vi "FilePath_Globals.vi"() -> ()   [LabVIEW 2019]
panel:
  in  "Flywheel Speeds File Path":string="/home/lvuser/autonomous/paths/"
  in  "Autonomous Paths File Path":string="/home/lvuser/autonomous/paths/"
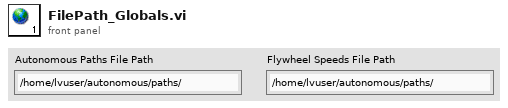
[diagram p1: front panel]
diagram:
